vi "sio ioctl.vi"(6 "parity":i32, 8 "stop bits":i32, 9 "data bits":i32, 10 "baud":i32, 11 "port":i32) -> (2 "port":i32, 3 "Status":i32)   [LabVIEW 2015, in "PCOMM.lvlib"]
doc: "int WINAPI sio_ioctl(int port, int baud, int mode);"
uses:
  PCOMM.lvlib
  PCOMM.DLL
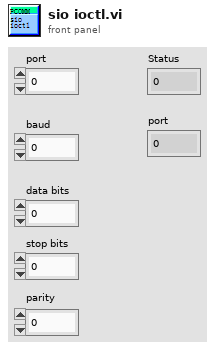
[diagram p1: front panel]
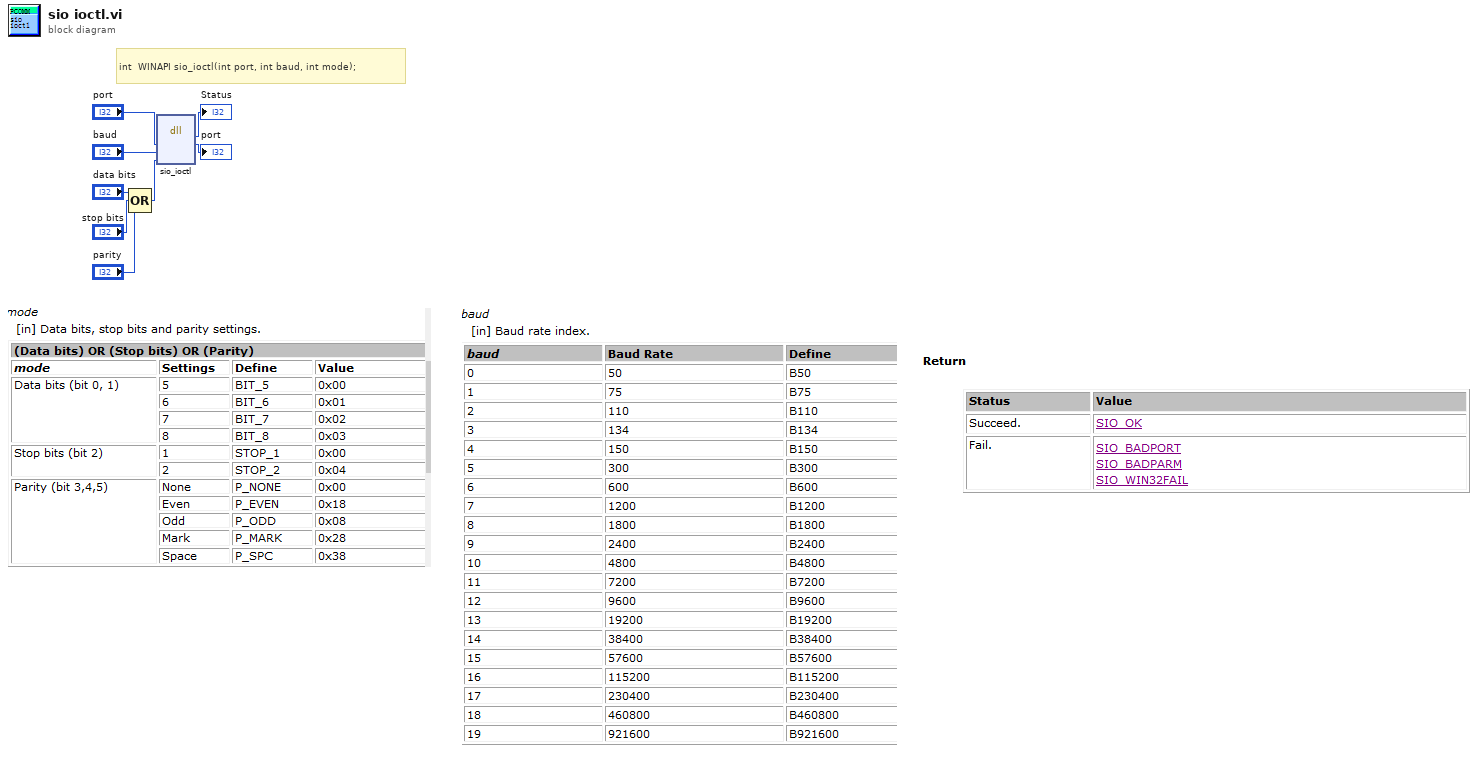
[diagram p0: block diagram]
diagram:
  # "int  WINAPI sio_ioctl(int port, int baud, int mode);"
  n1 = Compound Arithmetic op=OR ("复合运算")("data bits", "stop bits", "parity") -> (w2:i32)
  n2 = dll-call lib="PTH2^abs EDesktopLabview串口助手串口助手2.0Ing10_v3.2.0SubVIpcomm库PCOMM.*" fn="sio_ioctl"("port"="port", "baud"="baud", "mode"=w2) -> ("返回类型"=→"Status":i32, "port"=→"port":i32)  [unwired: 5 in, 2 out]
